vi "A Version Explorer - UI.vi"() -> ()   [LabVIEW 2020, in "A Version Explorer.lvlib"]
uses:
  A Version Explorer.lvlib
  Session/Session.lvclass
  <vilib>/Utility/miscctls.llb/LVRowAndColumnTypeDef.ctl
  Session/Session.lvclass/Session.ctl
  <userlib>/_OpenG.lib/file/file.llb/Valid Path - Traditional__ogtk.vi
  <userlib>/_OpenG.lib/array/array.llb/Index 1D Array Elements (String)__ogtk.vi
panel:
  in  "Project Folder":path
  in  "Select All/Some/None":enum8{"False", "True", "Mixed"}(c332)
  in  "Refresh":bool
  in  "Save for Previous Version":bool
  in  "LabVIEW Version":string
  in  "Files":i32[](listbox)
  out "Status":string
  in  "OK":bool
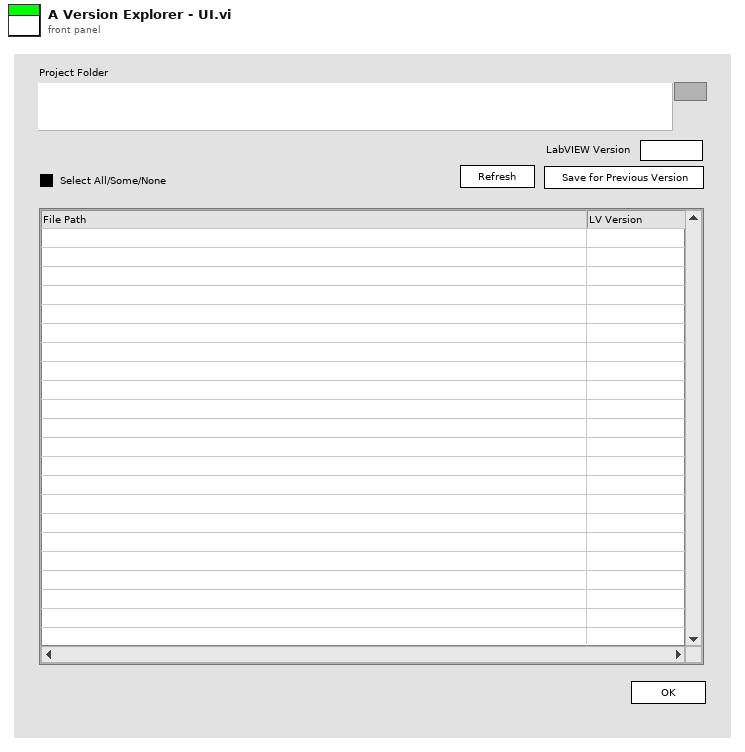
[diagram p1: front panel]
types:
  T1 = enum32{"Invalid", "Standard", "Closed", "Hidden", "Minimized", "Maximized"}
  T2 = enum32{"invalid app kind", "Development System", "Run Time System", "Student Edition", "Embedded LabVIEW", "Evaluation", "Custom"}
  T3 = typedef "LVRowAndColumnTypeDef.ctl" = cluster{"Row":i32, "Column":i32}
  T4 = typedef "eventvkey.ctl" = enum16{"ASCII", "Enter", "Return", "Shift", "Ctrl", "Alt", "Cmd", "Opt", "Caps", "NumLock", "Clear", "Break", "Up", "Down", "Left", "Right", "Insert", "Delete", "Home", "End", "PageUp", "PageDown", "Escape", "Help", "Pause", "ScrollLock", "F1", "F2", "F3", "F4", "F5", "F6", "F7", "F8", "F9", "F10", "F11", "F12", "F13", "F14", "F15", "F16", "F17", "F18", "F19", "F20", "F21", "F22", "F23", "F24", "Play", "VolumeUp", "VolumeDown", "Mute", "Two Byte Char"}
  T5 = cluster{"Shift":bool, "Ctrl":bool, "Alt":bool, "Cmd":bool, "Opt":bool}
  T6 = cluster{"Core":cluster{"Current VI Reference":refnum<vi>, "Close Panel on Exit?":bool}, "Your Boolean data":bool, "Session":refnum<class "Session.lvclass">}
  T7 = cluster{"Current VI Reference":refnum<vi>, "Close Panel on Exit?":bool}
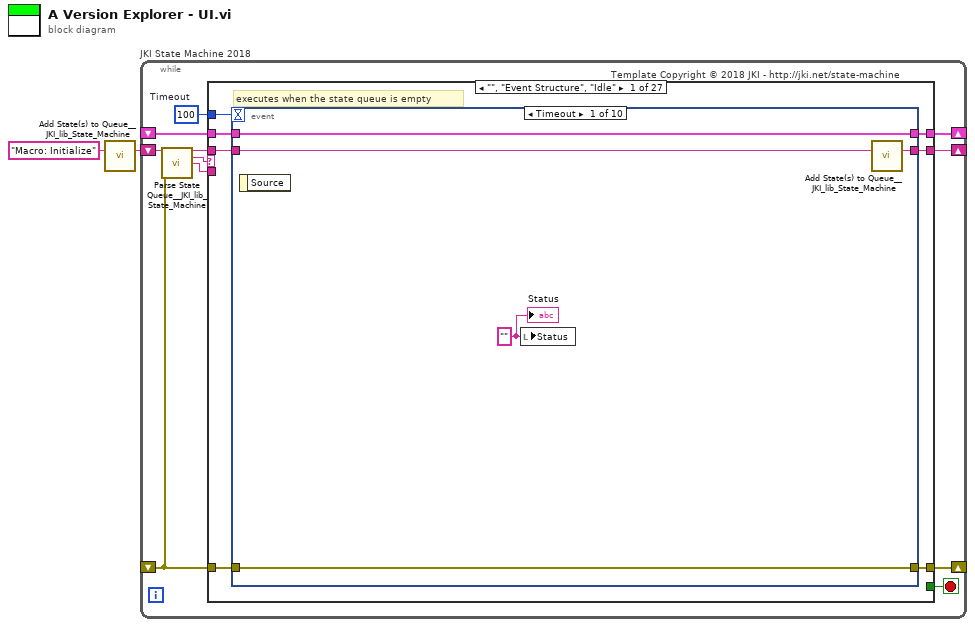
[diagram p0: block diagram]
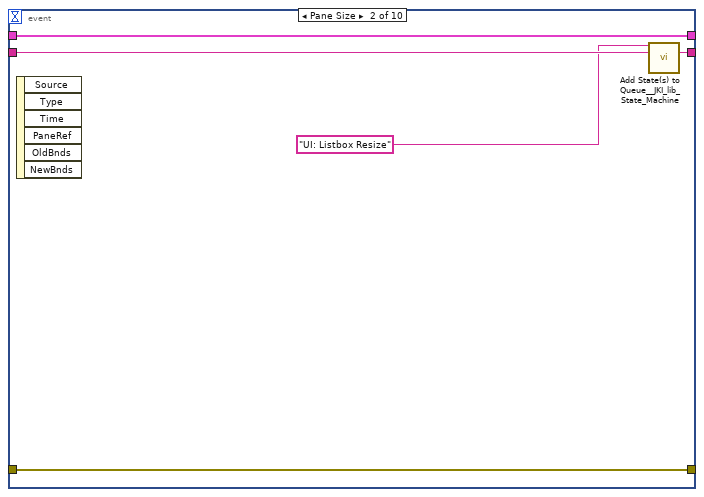
[diagram p2: hidden frame]
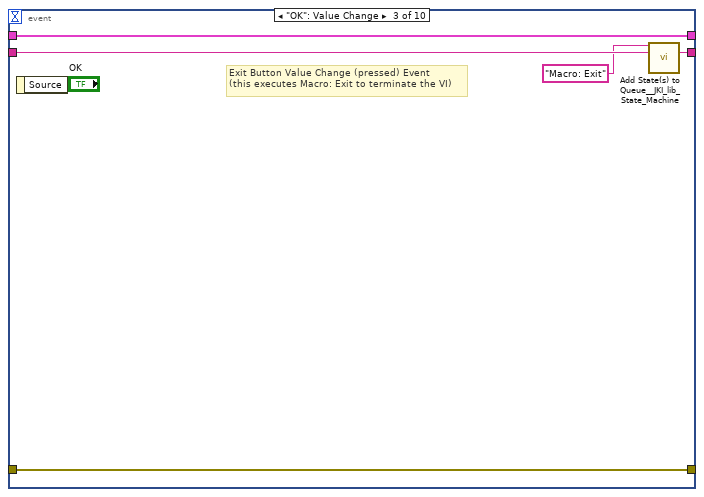
[diagram p3: hidden frame]
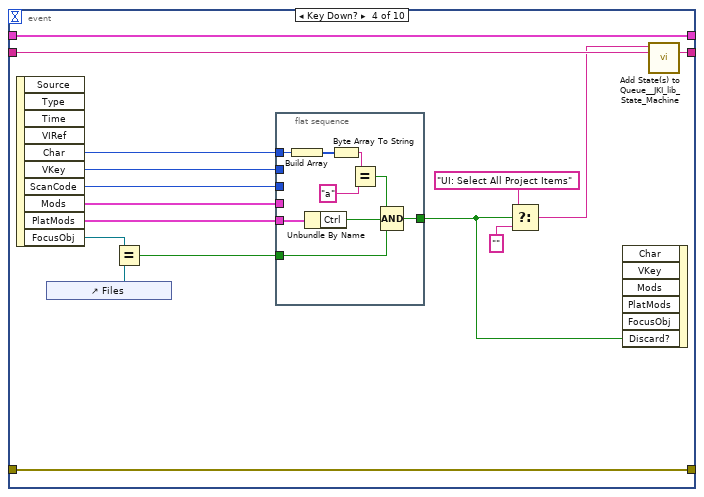
[diagram p4: hidden frame]
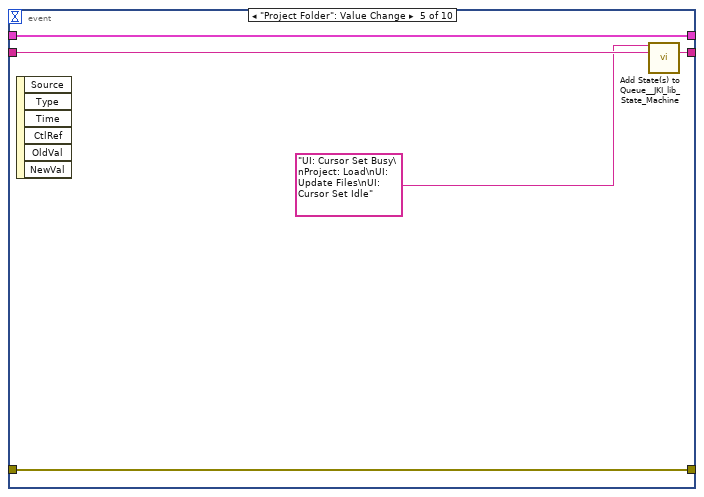
[diagram p5: hidden frame]
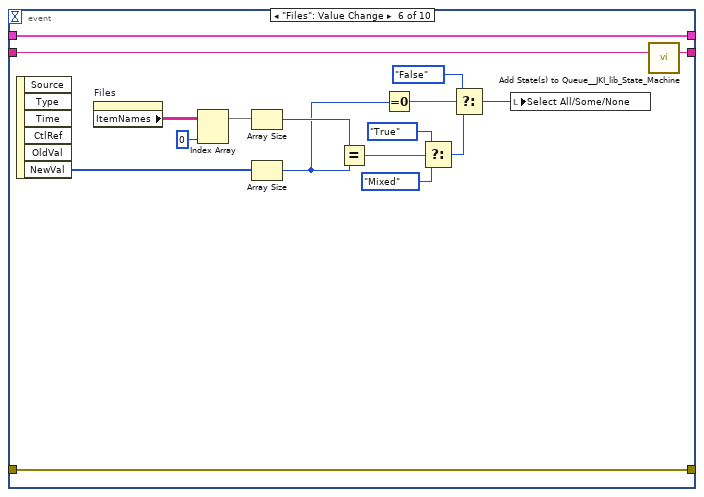
[diagram p6: hidden frame]
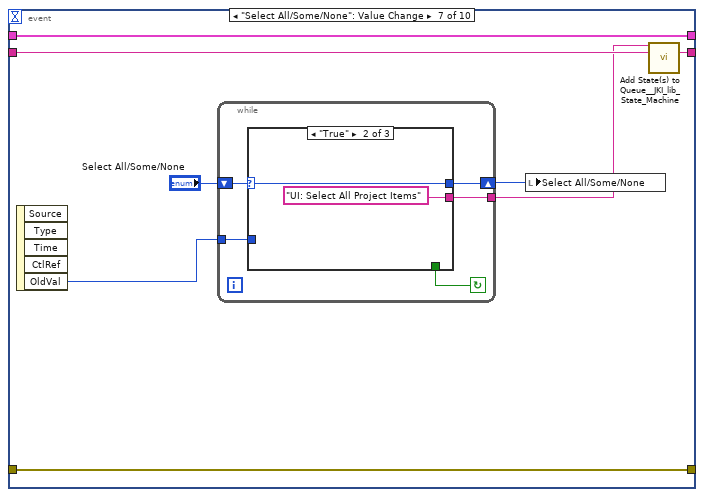
[diagram p7: hidden frame]
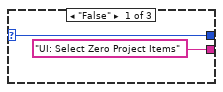
[diagram p8: hidden frame]
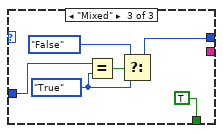
[diagram p9: hidden frame]
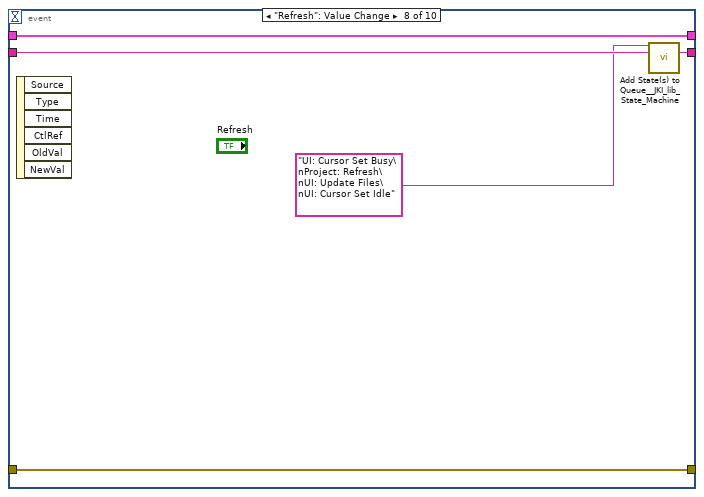
[diagram p10: hidden frame]
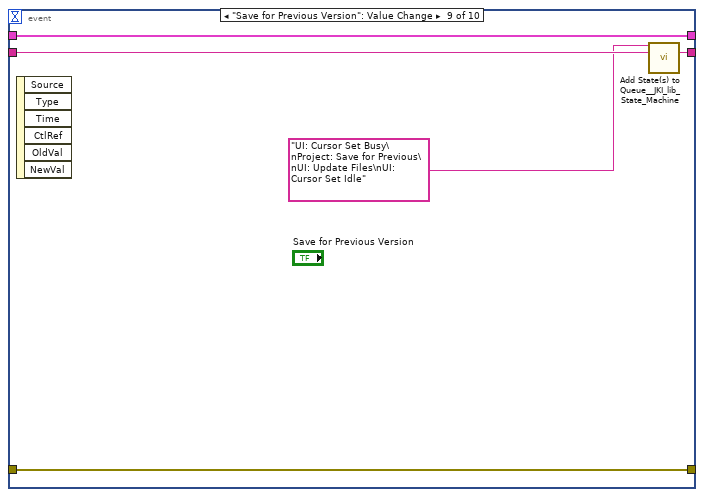
[diagram p11: hidden frame]
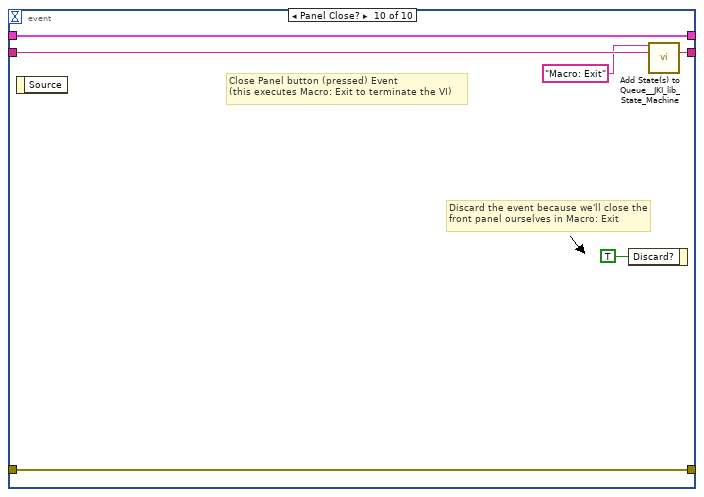
[diagram p12: hidden frame]
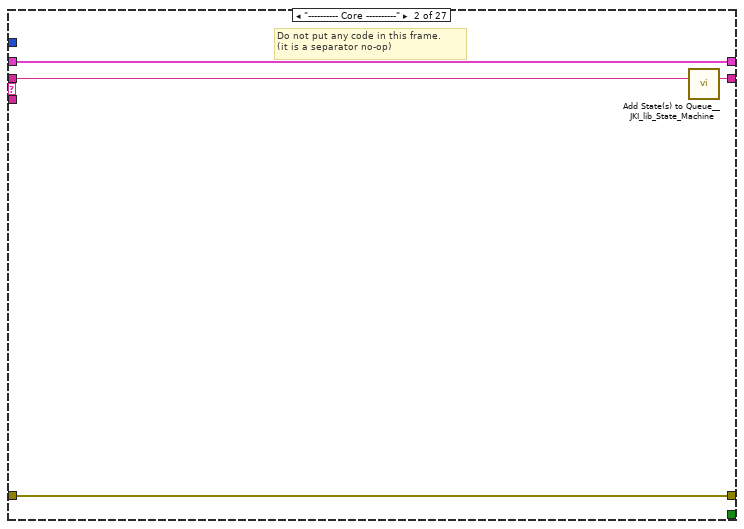
[diagram p13: hidden frame]
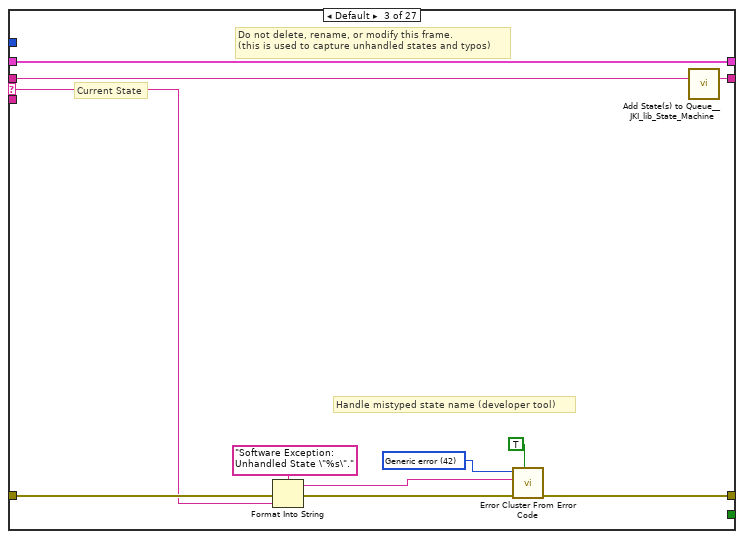
[diagram p14: hidden frame]
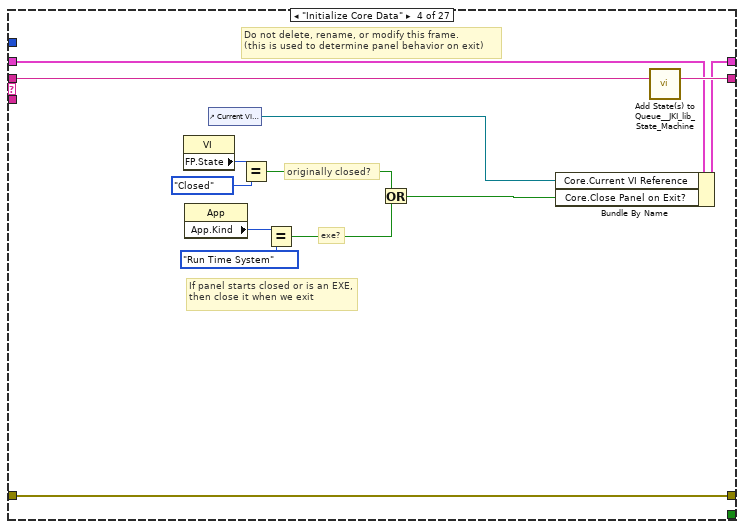
[diagram p15: hidden frame]
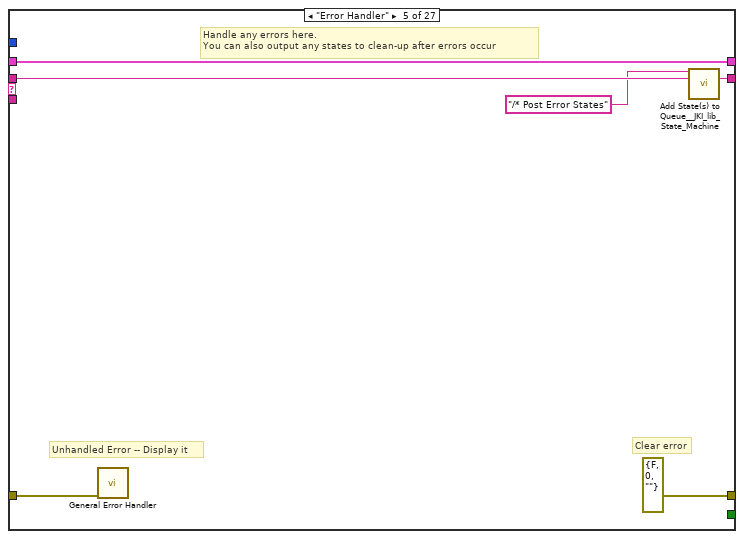
[diagram p16: hidden frame]
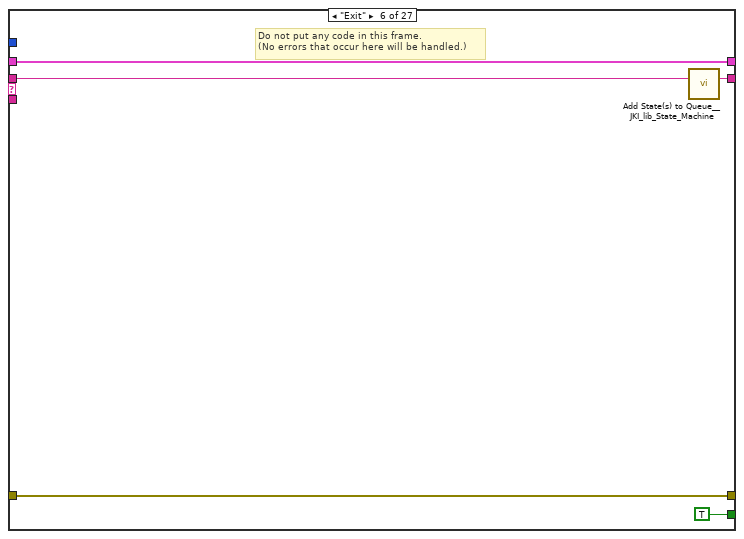
[diagram p17: hidden frame]
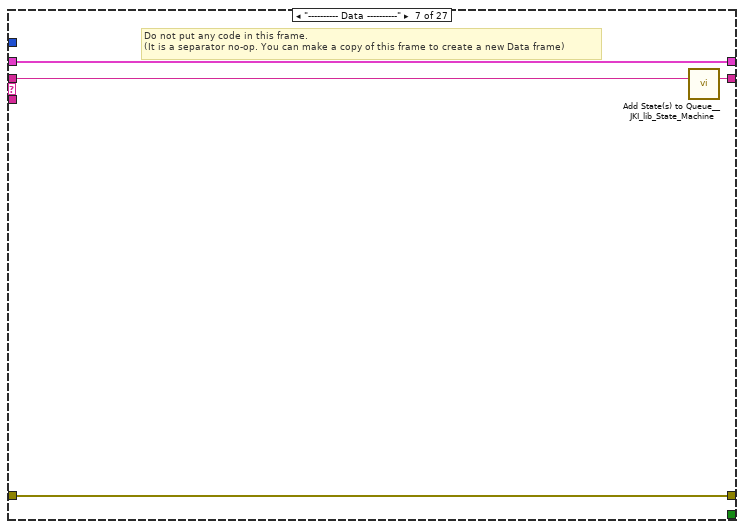
[diagram p18: hidden frame]
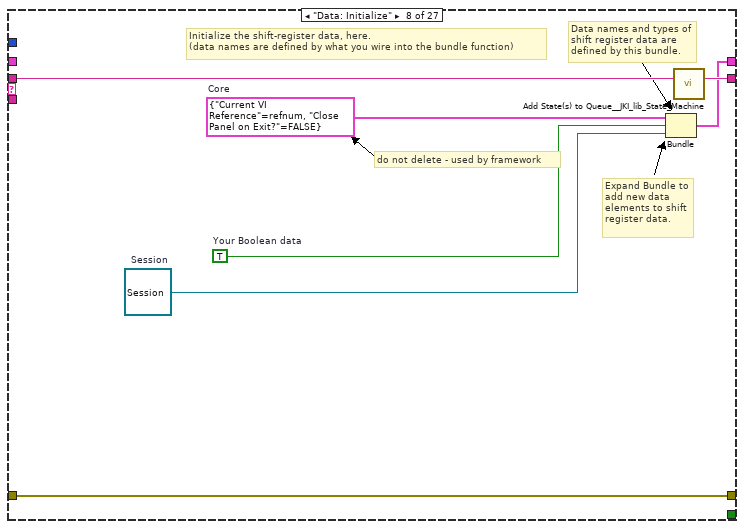
[diagram p19: hidden frame]
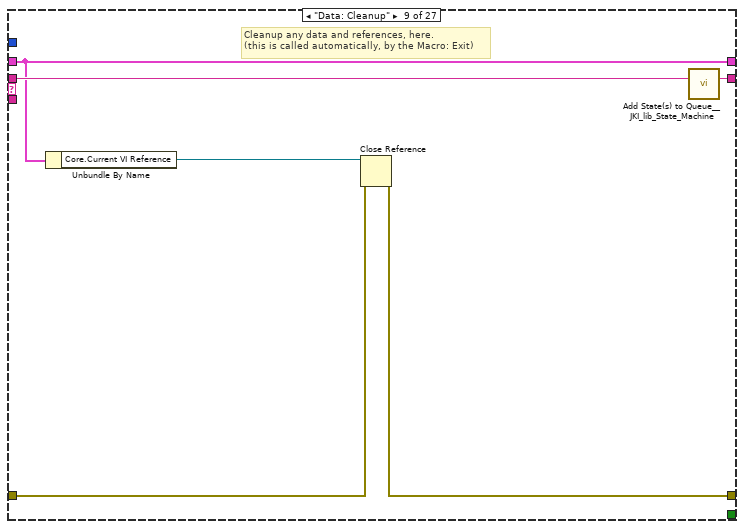
[diagram p20: hidden frame]
diagram:
  n1 = call <vilib>:"Add State(s) to Queue__JKI_lib_State_Machine.vi"("State(s) in (\"\")"="Macro: Initialize") -> ("States Out"=w2:string)  [unwired: 14 in]
  n2 = while "JKI State Machine 2018" {
    shift-right: [w6] -> _
    shift-left: _ -> [w5]
    shift-right: [w9] -> _
    shift-left: _ -> [w3]
    shift-right: [w8] -> _
    shift-left: w2 -> [w10]
    stop <- w7 stop-if-true
    w4 = 100  # Timeout
    # "Template Copyright © 2018 JKI - http://jki.net/state-machine"
    n3 = call <vilib>:"Parse State Queue__JKI_lib_State_Machine.vi"("State Queue"=w10, "Error In (no error)"=w3) -> ("Remaining States"=w12:string, "Current State"=w13:string, "Arguments"=w11:string)  [unwired: 11 in]
    n4 = case shown="\"\", \"Event Structure\", \"Idle\"" w13 {
      selector: w13 -> [_ _ w126 _ _ _ _ _ _ _ _ _ _ _ _ _ _ _ _ _ _ _ _ _ _ _ _]
      tunnel: w12 -> [w20 w125 w130 w149 w155 w160 w164 w171 w177 w181 w185 w189 w196 w203 w218 w223 w229 w239 w245 w256 w325 w335 w345 w349 w360 w369 w388]
      tunnel: w11 -> [_ _ _ _ _ _ _ _ _ _ _ _ _ _ _ _ _ _ w240 w250 _ _ _ _ _ _ _]
      tunnel: w5 -> [w18 w122 w128 w142 w152 w158 w161 _ w172 w178 w182 w186 w193 w200 w207 w221 w227 w237 w243 w252 w322 w332 w342 w347 w358 w363 w385]
      tunnel: [w17 w123 w132 w146 errorcluster {"status"=FALSE, "code"=0, "source"=""} ("error out") w157 w162 w168 w173 w179 w183 w187 w194 w201 w210 w220 w226 w236 w241 w253 w323 w333 w343 w346 w354 w365 w386] -> w9
      tunnel: w3 -> [w16 w123 w131 w146 w151 w157 w162 w168 w174 w179 w183 w187 w194 w201 w209 w220 w226 w236 w242 w254 w323 w333 w343 w346 w353 w366 w373]
      tunnel: [w19 w124 w129 w148 w154 w159 w163 w170 w176 w180 w184 w188 w195 w202 w217 w222 w228 w238 w244 w255 w324 w334 w344 w348 w359 w368 w387] -> w8
      tunnel: [_ _ _ _ _ TRUE _ _ _ _ _ _ _ _ _ _ _ _ _ _ _ _ _ _ _ _ _] -> w7
      tunnel: [w15 w122 w128 w147 w152 w158 w161 w169 w172 w178 w182 w186 w193 w200 w205 w221 w227 w237 w243 w252 w322 w332 w342 w347 w352 w367 w384] -> w6
      tunnel: w4 -> [w14 _ _ _ _ _ _ _ _ _ _ _ _ _ _ _ _ _ _ _ _ _ _ _ _ _ _]
      frame "", "Event Structure", "Idle" {
        # "executes when the state queue is empty"
        n5 = event shown="[0] Timeout" {
          selector: _ -> [_ _ _ _ _ _ _ _ _ _]
          dyn-events: _ -> [_ _ _ _ _ _ _ _ _ _]
          timeout: w14 -> [_ _ _ _ _ _ _ _ _ _]
          tunnel: w20 -> [w25 w30 w35 w51 w65 w82 w90 w110 w115 w121]
          tunnel: [w24 w29 w34 w50 w64 w81 w89 w109 w114 w120] -> w19
          tunnel: w18 -> [w22 w27 w32 w48 w62 w79 w87 w107 w112 w118]
          tunnel: [w23 w28 w33 w49 w63 w80 w88 w108 w113 w119] -> w17
          tunnel: w16 -> [w23 w28 w33 w49 w63 w80 w88 w108 w113 w119]
          tunnel: [w22 w27 w32 w48 w62 w79 w87 w107 w112 w118] -> w15
          event Timeout {
            w21 = "" ("Status")
            n6 = event-data() -> ()  [unwired: 1 in, 1 out]
            n7 = local write "Status"(w21) -> ()
            n8 = call <vilib>:"Add State(s) to Queue__JKI_lib_State_Machine.vi"("State(s) in (\"\")"=w25) -> ("States Out"=w24:string)  [unwired: 14 in]
            "Status" <- w21
          }
          event Pane Size {
            n9 = event-data() -> ()  [unwired: 1 in, 6 out]
            n10 = call <vilib>:"Add State(s) to Queue__JKI_lib_State_Machine.vi"("State(s) in Front (\"\")"="UI: Listbox Resize" ("Status"), "State(s) in (\"\")"=w30) -> ("States Out"=w29:string)  [unwired: 13 in]
          }
          event "OK": Value Change {
            # "Exit Button Value Change (pressed) Event\n(this executes Macro: Exit to terminate the VI)"
            n11 = event-data() -> ()  [unwired: 1 in, 1 out]
            n12 = call <vilib>:"Add State(s) to Queue__JKI_lib_State_Machine.vi"("State(s) in Front (\"\")"="Macro: Exit", "State(s) in (\"\")"=w35) -> ("States Out"=w34:string)  [unwired: 13 in]
          }
          event Key Down? {
            n13 = event-data() -> ("Char"=w41:i16, "VKey"=w42:T4, "ScanCode"=w43:i16, "Mods"=w47:cluster{"Num Pad":bool, "Menu Key":bool}, "PlatMods"=w46:T5, "FocusObj"=w45:refnum<vi>)  [unwired: 1 in, 4 out]
            n14 = control-ref of="Files"() -> (w44:refnum<vi>)
            n15 = Equal?(x=w45, y=w44) -> (x = y?=w40:bool)
            n16 = flat-sequence {
              tunnel: w47 -> [_]
              tunnel: w46 -> [w60]
              tunnel: w43 -> [_]
              tunnel: w42 -> [_]
              tunnel: w41 -> [w59]
              tunnel: w40 -> [w53]
              tunnel: [w52] -> w39
              frame #0 {
                n17 = Build Array(w59) -> (w58:i16[])
                n18 = Unbundle By Name(w60) -> ("Ctrl"=w54:bool)
                n19 = Byte Array To String(unsigned byte array=w58) -> (string=w57:string)
                n20 = Equal?(x=w57, y="a" ("string")) -> (x = y?=w55:bool)
                n21 = Compound Arithmetic op=AND(w55, w54, w53) -> (w52:bool)
              }
            }
            n22 = Select(t="UI: Select All Project Items", s=w39, f="") -> (s? t:f=w36:string)
            n23 = event-data("Discard?"=w39) -> ()  [unwired: 6 in, 1 out]
            n24 = call <vilib>:"Add State(s) to Queue__JKI_lib_State_Machine.vi"("State(s) in Front (\"\")"=w36, "State(s) in (\"\")"=w51) -> ("States Out"=w50:string)  [unwired: 13 in]
          }
          event "Project Folder": Value Change {
            n25 = event-data() -> ()  [unwired: 1 in, 6 out]
            n26 = call <vilib>:"Add State(s) to Queue__JKI_lib_State_Machine.vi"("State(s) in Front (\"\")"="UI: Cursor Set Busy\nProject: Load\nUI: Update Files\nUI: Cursor Set Idle", "State(s) in (\"\")"=w65) -> ("States Out"=w64:string)  [unwired: 13 in]
          }
          event "Files": Value Change {
            n27 = event-data() -> ("NewVal"=w77:i32[])  [unwired: 1 in, 5 out]
            n28 = property on="Files" class="MCListbox (strict)"() -> ("ItemNames"=w78:string[][])  [unwired: 2 in, 2 out]
            n29 = Index Array(array=w78, index (col)=0 ("disabled index (col)")) -> (element=w75:string[])  [unwired: 1 in]
            n30 = Array Size(array=w75) -> (size(s)=w76:i32)
            n31 = Array Size(array=w77) -> (size(s)=w73:i32)
            n32 = Equal?(x=w76, y=w73) -> (x = y?=w69:bool)
            n33 = Equal To 0?(x=w73) -> (x = 0?=w72:bool)
            n34 = Select(t=enum8{"False", "True", "Mixed"}."True" ("Select All/Some/None"), s=w69, f=enum8{"False", "True", "Mixed"}."Mixed" ("Select All/Some/None")) -> (s? t:f=w66:enum8{"False", "True", "Mixed"})
            n35 = Select(t=enum8{"False", "True", "Mixed"}."False" ("Select All/Some/None"), s=w72, f=w66) -> (s? t:f=w70:enum8{"False", "True", "Mixed"})
            n36 = local write "Select All/Some/None"(w70) -> ()
            n37 = call <vilib>:"Add State(s) to Queue__JKI_lib_State_Machine.vi"("State(s) in (\"\")"=w82) -> ("States Out"=w81:string)  [unwired: 14 in]
          }
          event "Select All/Some/None": Value Change {
            n38 = event-data() -> ("OldVal"=w84:enum8{"False", "True", "Mixed"})  [unwired: 1 in, 4 out]
            n39 = while {
              tunnel: [w94] -> w85
              tunnel: w84 -> [w93]
              shift-right: [w91] -> w83
              shift-left: "Select All/Some/None" -> [w95]
              stop <- w92 continue-if-true
              n40 = case shown="\"True\"" w95 {
                selector: w95 -> [w96 w98 _]
                tunnel: ["UI: Select Zero Project Items" "UI: Select All Project Items" _] -> w94
                tunnel: w93 -> [_ _ w104]
                tunnel: [_ _ TRUE] -> w92
                tunnel: [w96 w98 w100] -> w91
                frame "False" {
                }
                frame "True" {
                }
                frame "Mixed" {
                  w102 = enum8{"False", "True", "Mixed"}."True" ("Select All/Some/None")
                  n41 = Equal?(x=w104, y=w102) -> (x = y?=w103:bool)
                  n42 = Select(t=enum8{"False", "True", "Mixed"}."False" ("Select All/Some/None"), s=w103, f=w102) -> (s? t:f=w100:enum8{"False", "True", "Mixed"})
                }
              }
            }
            n43 = local write "Select All/Some/None"(w83) -> ()
            n44 = call <vilib>:"Add State(s) to Queue__JKI_lib_State_Machine.vi"("State(s) in Front (\"\")"=w85, "State(s) in (\"\")"=w90) -> ("States Out"=w89:string)  [unwired: 13 in]
          }
          event "Refresh": Value Change {
            n45 = event-data() -> ()  [unwired: 1 in, 6 out]
            n46 = call <vilib>:"Add State(s) to Queue__JKI_lib_State_Machine.vi"("State(s) in Front (\"\")"="UI: Cursor Set Busy\nProject: Refresh\nUI: Update Files\nUI: Cursor Set Idle", "State(s) in (\"\")"=w110) -> ("States Out"=w109:string)  [unwired: 13 in]
          }
          event "Save for Previous Version": Value Change {
            n47 = event-data() -> ()  [unwired: 1 in, 6 out]
            n48 = call <vilib>:"Add State(s) to Queue__JKI_lib_State_Machine.vi"("State(s) in Front (\"\")"="UI: Cursor Set Busy\nProject: Save for Previous\nUI: Update Files\nUI: Cursor Set Idle", "State(s) in (\"\")"=w115) -> ("States Out"=w114:string)  [unwired: 13 in]
          }
          event Panel Close? {
            # "Discard the event because we'll close the front panel ourselves in Macro: Exit"
            # "Close Panel button (pressed) Event\n(this executes Macro: Exit to terminate the VI)"
            n49 = event-data() -> ()  [unwired: 1 in, 1 out]
            n50 = event-data("Discard?"=TRUE) -> ()  [unwired: 1 in, 1 out]
            n51 = call <vilib>:"Add State(s) to Queue__JKI_lib_State_Machine.vi"("State(s) in Front (\"\")"="Macro: Exit", "State(s) in (\"\")"=w121) -> ("States Out"=w120:string)  [unwired: 13 in]
          }
        }
      }
      frame "---------- Core ----------" {
        # "Do not put any code in this frame.\n(it is a separator no-op)"
        n52 = call <vilib>:"Add State(s) to Queue__JKI_lib_State_Machine.vi"("State(s) in (\"\")"=w125) -> ("States Out"=w124:string)  [unwired: 14 in]
      }
      frame Default {
        w135 = 42 items=["No error", "Argument error", "Memory is full", "Out of zone", "End of file", "File already open", "Generic file I/O error", "File not found", "File permission error", "Disk is full", "Duplicate path", "Too many files open", "System feature not enabled", "Resource file not found", "Cannot add resource", "Resource not found", "Image not found", "Image memory error", "Pen does not exist", "Config type invalid", "Config token not found", "Config parse error", "Config memory error", "Bad external code format", "Bad external code offset", "External code not present", "Null window", "Destroy window error", "Null menu", "Print aborted", "Bad print record", "Print driver error", "Windows error during printing", "Memory error during printing", "Print dialog error", "Generic print error", "Invalid device refnum", "Device not found", "Device parameter error", "Device unit error", "Cannot open device", "Device call aborted", "Generic error", "Cancelled by user", "Object ID too low", "Object ID too high", "Object not in heap", "Unknown heap", "Unknown object (invalid DefProc)", "Unknown object (DefProc not in table)", "Message out of range", "Invalid (null) method", "Unknown message", "Manager call not supported", "Bad address", "Network operation in progress", "Network operation timed out", "Connection is busy", "Network attribute not supported", "Network error", "Address in use", "System out of memory", "Connection aborted", "Connection refused", "Not connected", "Already connected", "Connection closed", "Initialization error (interapplication manager)", "Bad occurrence", "Wait on unbound occurrence handler", "Occurrence queue overflow", "Datalog type conflict", "Unused", "Unrecognized type (interapplication manager)", "Memory corrupt", "Failed to make temporary DLL", "Old CIN version", "Drag socket not found", "Failed to load drop-object", "Failed to register OLE object", "Failed to release OLE object", "Format specifier type mismatch", "Unknown format specifier", "Too few format specifiers", "Too many format specifiers", "Scan failed", "Newer CIN version", "Error converting to variant", "Runtime menu error", "Password tampered", "Variant attribute not found", "Incompatible variant data type", "Event data is not available", "Event Store is not present", "Occurrence is not found", "Event Queue is not created", "Event info is not available", "Refnum passed is NULL", "Error retrieving Class GUID", "Error retrieving CoClass GUID", "Error retrieving TypeLib GUID.", "Bad built application magic bytes.", "Specific driver is different from the specific driver associated with the Logical Name.", "There is no session opened to the class driver.", "Max Error", "MAX - Error with config objects", "MAX - Error loading configuration", "MAX - Group not supported"]
        # "Current State"
        # "Do not delete, rename, or modify this frame.\n(this is used to capture unhandled states and typos)"
        # "Handle mistyped state name (developer tool)"
        n53 = Format Into String(format string="Software Exception: Unhandled State \"%s\"." ("message"), error in=w131, w126) -> (resulting string=w134:string, error out=w133:errorcluster)  [unwired: 1 in]
        n54 = call <vilib>:"Error Cluster From Error Code.vi"("show call chain? (False)"=TRUE, "error in (no error)"=w133, "error message (\"\")"=w134, "error code (0)"=w135) -> ("error out"=w132:errorcluster)  [unwired: 5 in]
        n55 = call <vilib>:"Add State(s) to Queue__JKI_lib_State_Machine.vi"("State(s) in (\"\")"=w130) -> ("States Out"=w129:string)  [unwired: 14 in]
      }
      frame "Initialize Core Data" {
        # "Do not delete, rename, or modify this frame.\n(this is used to determine panel behavior on exit)"
        # "originally closed?"
        # "exe?"
        # "If panel starts closed or is an EXE, then close it when we exit"
        n56 = property class="VI"() -> ("FP.State"=w139:T1)  [unwired: 2 in, 2 out]
        n57 = property class="App"() -> ("App.Kind"=w145:T2)  [unwired: 2 in, 2 out]
        n58 = control-ref of="Current VI Reference"() -> (w140:refnum<vi>)
        n59 = Equal?(x=w139, y=T1."Closed" ("Front Panel Window:State")) -> (x = y?=w137:bool)
        n60 = Equal?(x=w145, y=T2."Run Time System" ("Application:Kind")) -> (x = y?=w143:bool)
        n61 = Or(x=w137, y=w143) -> (x .or. y?=w141:bool)
        n62 = Bundle By Name(cluster=w142, "Core.Current VI Reference"=w140, "Core.Close Panel on Exit?"=w141) -> (w147:T6)
        n63 = call <vilib>:"Add State(s) to Queue__JKI_lib_State_Machine.vi"("State(s) in (\"\")"=w149) -> ("States Out"=w148:string)  [unwired: 14 in]
      }
      frame "Error Handler" {
        # "Unhandled Error -- Display it"
        # "Handle any errors here.\nYou can also output any states to clean-up after errors occur"
        # "Clear error"
        n64 = call <vilib>:"General Error Handler.vi"("error in (no error)"=w151) -> ()  [unwired: 10 in, 5 out]
        n65 = call <vilib>:"Add State(s) to Queue__JKI_lib_State_Machine.vi"("State(s) in Front (\"\")"="/* Post Error States", "State(s) in (\"\")"=w155) -> ("States Out"=w154:string)  [unwired: 13 in]
      }
      frame "Exit" {
        # "Do not put any code in this frame.\n(No errors that occur here will be handled.)"
        n66 = call <vilib>:"Add State(s) to Queue__JKI_lib_State_Machine.vi"("State(s) in (\"\")"=w160) -> ("States Out"=w159:string)  [unwired: 14 in]
      }
      frame "---------- Data ----------" {
        # "Do not put any code in this frame.\n(It is a separator no-op. You can make a copy of this frame to create a new Data frame)"
        n67 = call <vilib>:"Add State(s) to Queue__JKI_lib_State_Machine.vi"("State(s) in (\"\")"=w164) -> ("States Out"=w163:string)  [unwired: 14 in]
      }
      frame "Data: Initialize" {
        w165 = refnum<class "Session.lvclass"> refnum  # Session
        w166 = T7 {"Current VI Reference"=refnum, "Close Panel on Exit?"=FALSE}  # Core
        w167 = TRUE  # Your Boolean data
        # "do not delete - used by framework"
        # "Expand Bundle to add new data elements to shift register data."
        # "Data names and types of shift register data are defined by this bundle."
        # "Initialize the shift-register data, here.\n(data names are defined by what you wire into the bundle function)"
        n68 = Bundle("Core"=w166, "Your Boolean data"=w167, "Session"=w165) -> (w169:T6)  [unwired: 1 in]
        n69 = call <vilib>:"Add State(s) to Queue__JKI_lib_State_Machine.vi"("State(s) in (\"\")"=w171) -> ("States Out"=w170:string)  [unwired: 14 in]
      }
      frame "Data: Cleanup" {
        # "Cleanup any data and references, here.\n(this is called automatically, by the Macro: Exit)"
        n70 = Unbundle By Name(w172) -> ("Core.Current VI Reference"=w175:refnum<vi>)
        n71 = Close Reference(reference=w175, error in (no error)=w174) -> (error out=w173:errorcluster)
        n72 = call <vilib>:"Add State(s) to Queue__JKI_lib_State_Machine.vi"("State(s) in (\"\")"=w177) -> ("States Out"=w176:string)  [unwired: 14 in]
      }
      frame "---------- UI ----------" {
        # "Do not put any code in this frame.\n(It is a separator no-op. You can make a copy of this frame to create a new UI frame)"
        n73 = call <vilib>:"Add State(s) to Queue__JKI_lib_State_Machine.vi"("State(s) in (\"\")"=w181) -> ("States Out"=w180:string)  [unwired: 14 in]
      }
      frame "UI: Cursor Set Busy" {
        # "Do not put any code in this frame.\n(It is a separator no-op. You can make a copy of this frame to create a new UI frame)"
        n74 = call <vilib>:"Set Busy.vi"() -> ()  [unwired: 10 in, 2 out]
        n75 = call <vilib>:"Add State(s) to Queue__JKI_lib_State_Machine.vi"("State(s) in (\"\")"=w185) -> ("States Out"=w184:string)  [unwired: 14 in]
      }
      frame "UI: Cursor Set Idle" {
        # "Do not put any code in this frame.\n(It is a separator no-op. You can make a copy of this frame to create a new UI frame)"
        n76 = call <vilib>:"Unset Busy.vi"() -> ()  [unwired: 11 in, 1 out]
        n77 = call <vilib>:"Add State(s) to Queue__JKI_lib_State_Machine.vi"("State(s) in (\"\")"=w189) -> ("States Out"=w188:string)  [unwired: 14 in]
      }
      frame "UI: Select All Project Items" {
        # "Do not put any code in this frame.\n(It is a separator no-op. You can make a copy of this frame to create a new UI frame)"
        n78 = property on="Files" class="MCListbox (strict)"() -> ("ItemNames"=w192:string[][])  [unwired: 2 in, 2 out]
        n79 = local write "Select All/Some/None"(enum8{"False", "True", "Mixed"}."True" ("Select All/Some/None")) -> ()
        n80 = for {
          tunnel: w192 -> [_] mode=indexing
          tunnel: [w197] -> w191 mode=indexing
          i -> [w197]
        }
        n81 = property on="Files" class="MCListbox (strict)"("Value"=w191) -> ()  [unwired: 2 in, 2 out]
        n82 = call <vilib>:"Add State(s) to Queue__JKI_lib_State_Machine.vi"("State(s) in (\"\")"=w196) -> ("States Out"=w195:string)  [unwired: 14 in]
      }
      frame "UI: Select Zero Project Items" {
        n83 = local write "Select All/Some/None"(enum8{"False", "True", "Mixed"}."False" ("Select All/Some/None")) -> ()
        n84 = property on="Files" class="MCListbox (strict)"("Value"=i32[] [] ("Files")) -> ()  [unwired: 2 in, 2 out]
        n85 = call <vilib>:"Add State(s) to Queue__JKI_lib_State_Machine.vi"("State(s) in (\"\")"=w203) -> ("States Out"=w202:string)  [unwired: 14 in]
      }
      frame "UI: Update Files" {
        w211 = TRUE  # relative paths
        n86 = Unbundle By Name(w207) -> ("Session"=w206:refnum<class "Session.lvclass">)
        n87 = call "Get File Paths and Versions.vi"("relative paths? (F: Absolute)"=w211, "error in (no error)"=w209, "Session in"=w206) -> ("error out"=w210:errorcluster, "Versions"=w213:string[], "File Paths"=w215:path[], "Session out"=w204:refnum<class "Session.lvclass">)  [unwired: 5 in]
        n88 = Bundle By Name(cluster=w207, "Session"=w204) -> (w205:T6)
        n89 = Path To String(path=w215) -> (string=w214:string[])
        n90 = Build Array(w214, w213) -> (w212:string[][])
        n91 = Transpose 2D Array(2D array=w212) -> (transposed array=w208:string[][])
        n92 = property on="Files" class="MCListbox (strict)"("ColHdrString"=string[] ["File Path", "LV Version"] ("Row Header Strings[]"), "ItemNames"=w208) -> ()  [unwired: 2 in, 2 out]
        n93 = call <vilib>:"Add State(s) to Queue__JKI_lib_State_Machine.vi"("State(s) in (\"\")"=w218) -> ("States Out"=w217:string)  [unwired: 14 in]
      }
      frame "UI: Initialize" {
        # "Initialize the User Interface, here.\n(this is called automatically, by the Macro: Init)"
        n94 = local write "Status"("" ("Status")) -> ()
        n95 = call <vilib>:"Add State(s) to Queue__JKI_lib_State_Machine.vi"("State(s) in (\"\")"=w223) -> ("States Out"=w222:string)  [unwired: 14 in]
      }
      frame "UI: Uninitialize" {
        n96 = local write "Status"("" ("Status")) -> ()
        n97 = property on="Files" class="MCListbox (strict)"("ItemNames"=string[][] [] ("Item Names")) -> ()  [unwired: 2 in, 2 out]
        n98 = call <vilib>:"Add State(s) to Queue__JKI_lib_State_Machine.vi"("State(s) in (\"\")"=w229) -> ("States Out"=w228:string)  [unwired: 14 in]
      }
      frame "UI: Listbox Resize" {
        w231 = 100 ("y")
        n99 = property on="Files" class="MCListbox (strict)"() -> ("ContentRectBoundsWidth"=w233:i32)  [unwired: 2 in, 2 out]
        n100 = Subtract(x=w233, y=w231) -> (x-y=w234:i32)
        n101 = property on="Files" class="MCListbox (strict)"("ActiveCell"=T3 {"Row"=-2, "Column"=0} ("Active Cell:Active Cell"), "Width"=w234) -> (error out=w235:errorcluster)  [unwired: 2 in, 1 out]
        n102 = property on="Files" class="MCListbox (strict)"(error in=w235, "ActiveCell"=T3 {"Row"=-2, "Column"=1} ("Active Cell:Active Cell"), "Width"=w231) -> ()  [unwired: 1 in, 2 out]
        n103 = call <vilib>:"Add State(s) to Queue__JKI_lib_State_Machine.vi"("State(s) in (\"\")"=w239) -> ("States Out"=w238:string)  [unwired: 14 in]
      }
      frame "UI: Cursor Set" {
        # "Argument"
        # "Set and Unset Cursor Busy.\n(Usage: \"UI: Cursor Set >> Busy|Idle\")"
        n104 = case shown="\"Idle\", Default" w240 {
          tunnel: w242 -> [w247 w249]
          tunnel: [w246 w248] -> w241
          frame "Idle", Default {
            n105 = call <vilib>:"Unset Busy.vi"("error in (no error)"=w247) -> ("error out"=w246:errorcluster)  [unwired: 10 in]
          }
          frame "Busy" {
            n106 = call <vilib>:"Set Busy.vi"("error in (no error)"=w249) -> ("error out"=w248:errorcluster)  [unwired: 9 in, 1 out]
          }
        }
        n107 = call <vilib>:"Add State(s) to Queue__JKI_lib_State_Machine.vi"("State(s) in (\"\")"=w245) -> ("States Out"=w244:string)  [unwired: 14 in]
      }
      frame "UI: Front Panel State" {
        # "Argument"
        # "Set Front Panel Open or Closed\n(Usage: \"UI: Front Panel State >> Open|Close\")"
        n108 = Unbundle By Name(w252) -> ("Core.Current VI Reference"=w251:refnum<vi>)
        n109 = case shown="\"Minimize\", \"Minimized\"" w250 {
          tunnel: w254 -> [w262 w277 w288 w301 w314]
          tunnel: [w264 w278 w290 w303 w316] -> w253
          tunnel: w251 -> [w263 w275 w289 w302 w315]
          frame "Open", "Standard", Default {
            w257 = T1."Standard" ("State")
            n110 = property class="VI"(reference=w263, error in=w262) -> (reference out=w260:refnum<vi>, error out=w261:errorcluster, "FP.State"=w259:T1)
            n111 = Not Equal?(x=w259, y=w257) -> (x != y?=w258:bool)
            n112 = case shown="True" w258 {
              tunnel: [w268 w270] -> w264
              tunnel: w261 -> [w267 w270]
              tunnel: w260 -> [w266 _]
              tunnel: w257 -> [w265 _]
              frame True {
                n113 = invoke class="VI" method="FP.Open"(reference=w266, error in=w267, "Activate"=TRUE, "State"=w265) -> (error out=w268:errorcluster)  [unwired: 1 in, 4 out]
              }
              frame False {
              }
            }
          }
          frame "Close", "Closed" {
            n114 = property class="VI"(reference=w275, error in=w277) -> (reference out=w274:refnum<vi>, error out=w276:errorcluster, "FP.State"=w272:T1)
            n115 = Not Equal?(x=w272, y=T1."Closed" ("Front Panel Window:State")) -> (x != y?=w271:bool)
            n116 = case shown="True" w271 {
              tunnel: [w279 w282] -> w278
              tunnel: w276 -> [w279 w281]
              tunnel: w274 -> [_ w280]
              frame False {
              }
              frame True {
                n117 = invoke class="VI" method="FP.Close"(reference=w280, error in=w281) -> (error out=w282:errorcluster)  [unwired: 1 in, 2 out]
              }
            }
          }
          frame "Hidden", "Hide" {
            w283 = T1."Hidden" ("State")
            n118 = property class="VI"(reference=w289, error in=w288) -> (reference out=w286:refnum<vi>, error out=w287:errorcluster, "FP.State"=w285:T1)
            n119 = Not Equal?(x=w285, y=w283) -> (x != y?=w284:bool)
            n120 = case shown="True" w284 {
              tunnel: [w294 w295] -> w290
              tunnel: w287 -> [w293 w295]
              tunnel: w286 -> [w292 _]
              tunnel: w283 -> [w291 _]
              frame True {
                n121 = invoke class="VI" method="FP.Open"(reference=w292, error in=w293, "State"=w291) -> (error out=w294:errorcluster)  [unwired: 2 in, 4 out]
              }
              frame False {
              }
            }
          }
          frame "Minimize", "Minimized" {
            w296 = T1."Minimized" ("State")
            n122 = property class="VI"(reference=w302, error in=w301) -> (reference out=w299:refnum<vi>, error out=w300:errorcluster, "FP.State"=w298:T1)
            n123 = Not Equal?(x=w298, y=w296) -> (x != y?=w297:bool)
            n124 = case shown="True" w297 {
              tunnel: [w307 w308] -> w303
              tunnel: w300 -> [w306 w308]
              tunnel: w299 -> [w305 _]
              tunnel: w296 -> [w304 _]
              frame True {
                n125 = invoke class="VI" method="FP.Open"(reference=w305, error in=w306, "State"=w304) -> (error out=w307:errorcluster)  [unwired: 2 in, 4 out]
              }
              frame False {
              }
            }
          }
          frame "Maximize", "Maximized" {
            w309 = T1."Maximized" ("State")
            n126 = property class="VI"(reference=w315, error in=w314) -> (reference out=w312:refnum<vi>, error out=w313:errorcluster, "FP.State"=w311:T1)
            n127 = Not Equal?(x=w311, y=w309) -> (x != y?=w310:bool)
            n128 = case shown="True" w310 {
              tunnel: [w320 w321] -> w316
              tunnel: w313 -> [w319 w321]
              tunnel: w312 -> [w318 _]
              tunnel: w309 -> [w317 _]
              frame True {
                n129 = invoke class="VI" method="FP.Open"(reference=w318, error in=w319, "State"=w317) -> (error out=w320:errorcluster)  [unwired: 2 in, 4 out]
              }
              frame False {
              }
            }
          }
        }
        n130 = call <vilib>:"Add State(s) to Queue__JKI_lib_State_Machine.vi"("State(s) in (\"\")"=w256) -> ("States Out"=w255:string)  [unwired: 14 in]
      }
      frame "---------- Macro ----------" {
        # "Do not put any code in this frame.\n(It is a separator no-op. You can make a copy of this frame to create a new Macro frame)"
        n131 = call <vilib>:"Add State(s) to Queue__JKI_lib_State_Machine.vi"("State(s) in (\"\")"=w325) -> ("States Out"=w324:string)  [unwired: 14 in]
      }
      frame "Macro: Initialize" {
        w331 = "Data: Initialize\nInitialize Core Data\nUI: Initialize\nUI: Select Zero Project Items\nUI: Listbox Resize\nUI: Front Panel State >> Open"  # Data: Initialize Initialize Core Data UI: Initialize UI: Select Zero Project Items UI: Listbox Resize UI: Front Panel State >> Open
        # "Initialization Macro\n(This is called once, when the VI starts)"
        n132 = local read "Project Folder"() -> (w330:path)
        n133 = call-poly <userlib>:"Valid Path__ogtk.vi"("path"=w330) -> ("valid"=w329:bool)
        n134 = Select(t="Project: Load\nUI: Update Files", s=w329, f="") -> (s? t:f=w326:string)
        n135 = call <vilib>:"Add State(s) to Queue__JKI_lib_State_Machine.vi"("State(s) in Front (\"\")"=w331, "State(s) in (\"\")"=w335, "State(s) at Back (\"\")"=w326) -> ("States Out"=w334:string)  [unwired: 12 in]
      }
      frame "Macro: Exit" {
        # "Exit Macro\n(This is called once, when the VI exits)"
        n136 = Unbundle By Name(w342) -> ("Core.Close Panel on Exit?"=w341:bool)
        n137 = Select(t="UI: Front Panel State >> Close", s=w341, f="") -> (s? t:f=w338:string)
        n138 = call <vilib>:"Add State(s) to Queue__JKI_lib_State_Machine.vi"("State(s) in (\"\")"=w338, "State(s) at Back (\"\")"="UI: Uninitialize\nData: Cleanup\nExit") -> ("States Out"=w336:string)  [unwired: 13 in]
        n139 = call <vilib>:"Add State(s) to Queue__JKI_lib_State_Machine.vi"("State(s) in Front (\"\")"=w336, "State(s) in (\"\")"=w345) -> ("States Out"=w344:string)  [unwired: 13 in]
      }
      frame "---------- Project ----------" {
        n140 = call <vilib>:"Add State(s) to Queue__JKI_lib_State_Machine.vi"("State(s) in (\"\")"=w349) -> ("States Out"=w348:string)  [unwired: 14 in]
      }
      frame "Project: Load" {
        n141 = call "Create.vi"("error in (no error)"=w353, "Source Folder"="Project Folder") -> ("error out"=w356:errorcluster, "Session out"=w357:refnum<class "Session.lvclass">)  [unwired: 8 in]
        n142 = local write "Status"("Loading Project" ("Status")) -> ()
        n143 = call "Add Folder Recursively.vi"("error in (no error)"=w356, "Folder"="Project Folder", "Session in"=w357) -> ("error out"=w354:errorcluster, "Session out"=w351:refnum<class "Session.lvclass">)  [unwired: 7 in]
        n144 = Bundle By Name(cluster=w358, "Session"=w351) -> (w352:T6)
        n145 = call <vilib>:"Add State(s) to Queue__JKI_lib_State_Machine.vi"("State(s) in (\"\")"=w360) -> ("States Out"=w359:string)  [unwired: 14 in]
      }
      frame "Project: Refresh" {
        n146 = Unbundle By Name(w363) -> ("Session"=w362:refnum<class "Session.lvclass">)
        n147 = call "Refresh Files Info.vi"("error in (no error)"=w366, "Session in"=w362) -> ("error out"=w365:errorcluster, "Session out"=w364:refnum<class "Session.lvclass">)  [unwired: 8 in]
        n148 = local write "Status"("Reloading Project" ("Status")) -> ()
        n149 = Bundle By Name(cluster=w363, "Session"=w364) -> (w367:T6)
        n150 = call <vilib>:"Add State(s) to Queue__JKI_lib_State_Machine.vi"("State(s) in (\"\")"=w369) -> ("States Out"=w368:string)  [unwired: 14 in]
      }
      frame "Project: Save for Previous" {
        n151 = property on="Files" class="MCListbox (strict)"() -> ("ItemNames"=w380:string[][], "Value"=w382:i32[])  [unwired: 2 in, 2 out]
        n152 = Index Array(array=w380, index (col)=0 ("disabled index (col)")) -> (element=w379:string[])  [unwired: 1 in]
        n153 = Unbundle By Name(w385) -> ("Session"=w376:refnum<class "Session.lvclass">)
        n154 = call-poly <userlib>:"Index Array Elements__ogtk.vi"("indices"=w382, "array"=w379) -> ("elements"=w378:string[])  [unwired: 9 in]
        n155 = String To Path(string=w378) -> (path=w377:path[])
        n156 = call "Write LabVIEW Version.vi"("error in (no error)"=w373, "LabVIEW Version"="LabVIEW Version", "Session in"=w376) -> ("error out"=w374:errorcluster, "Session out"=w375:refnum<class "Session.lvclass">)  [unwired: 7 in]
        n157 = Format Into String(format string="Saving Project Files for LabVIEW %s" ("Status"), "LabVIEW Version") -> (resulting string=w371:string)  [unwired: 2 in, 1 out]
        n158 = call "Save Files for Previous Version.vi"("error in (no error)"=w374, "LabVIEW Files to Convert"=w377, "Session in"=w375) -> ("error out"=w386:errorcluster, "Session out"=w383:refnum<class "Session.lvclass">)  [unwired: 7 in]
        n159 = local write "Status"(w371) -> ()
        n160 = Bundle By Name(cluster=w385, "Session"=w383) -> (w384:T6)
        n161 = call <vilib>:"Add State(s) to Queue__JKI_lib_State_Machine.vi"("State(s) in (\"\")"=w388) -> ("States Out"=w387:string)  [unwired: 14 in]
      }
    }
  }
